vi "supprimerdonneeuser.vi"(0 "Validation":bool, 1 "AdminPassword":string, 2 "Identifiant":string, 3 "Fichier DB":string) -> ()   [LabVIEW 2024]
uses:
  <vilib>/drjdpowell/SQLite Library/SQL Connection/Open (string).vi
  <vilib>/drjdpowell/SQLite Library/SQL Connection/Execute SQL (No results).vi
  <vilib>/drjdpowell/SQLite Library/SQL Connection/Connection.lvclass
  <vilib>/drjdpowell/SQLite Library/SQLite.lvlib
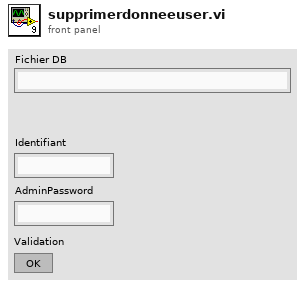
[diagram p1: front panel]
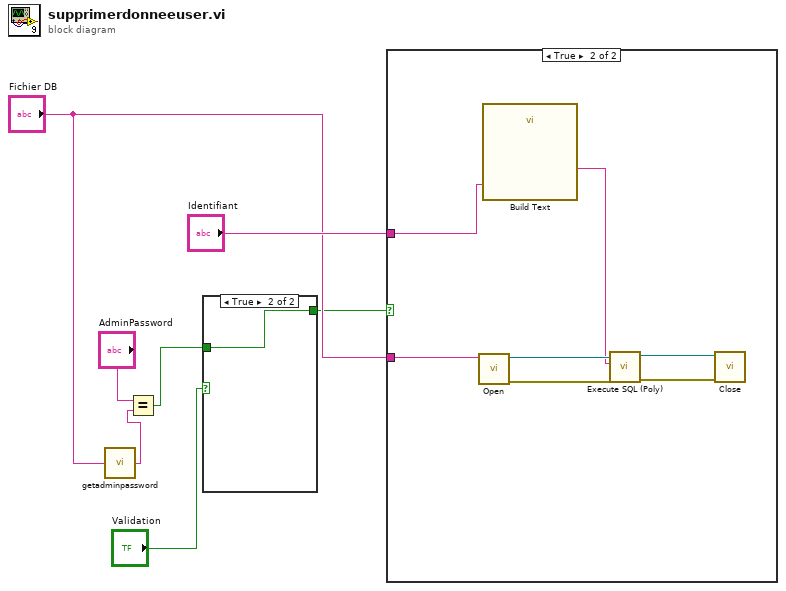
[diagram p0: block diagram]
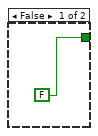
[diagram p2: hidden frame]
diagram:
  n1 = call "getadminpassword.vi"("Fichier DB"="Fichier DB") -> ("Password"=w5:string)
  n2 = Equal?(x="AdminPassword", y=w5) -> (x = y?=w1:bool)
  n3 = case shown="True" "Validation" {
    tunnel: [FALSE w9] -> w2
    tunnel: w1 -> [_ w9]
    frame False {
    }
    frame True {
    }
  }
  n4 = case shown="True" w2 {
    tunnel: "Fichier DB" -> [_ w11]
    tunnel: "Identifiant" -> [_ w10]
    frame False {
    }
    frame True {
      n5 = call-poly <vilib>:"Open.vi"("db file"=w11) -> ("error out"=w15:errorcluster, "SQLite Connection"=w16:refnum<class "Connection.lvclass">)  [unwired: 9 in]
      n6 = call "Build Text"("id"=w10) -> ("Result"=w14:string)  [unwired: 13 in, 1 out]
      n7 = call-poly <vilib>:"Execute SQL (Poly).vi"("error in (no error)"=w15, "SQL"=w14, "SQLite Connection in"=w16) -> ("error out"=w13:errorcluster, "SQLite Connection"=w12:refnum<class "Connection.lvclass">)  [unwired: 7 in]
      n8 = call-dynamic "Close.vi"("error in (no error)"=w13, "SQLite Connection in"=w12) -> ()  [unwired: 9 in, 1 out]
    }
  }
